vi "Write Data.vi"(7 "Address":u16=65535 format="%.0x", 8 "error in (no error)":errorcluster, 9 "Data":i32[](array[numeric]), 10 "Specified Num in":u8=1, 11 "Port Selection Info":T1={"Port Name"="", "Amplifier Num"=1, "Baud Rate"=38400, "Char Formation"=enum."0"} {"Baud Rate" items=["38400"=38400, "19200"=19200, "9600"=9600, "115200"=0]; "Amplifier Num" max=31}) -> (0 "error out":errorcluster, 2 "Specified Num out":u8=1, 3 "Port Selection Info Out":T1={"Port Name"="", "Amplifier Num"=1, "Baud Rate"=38400, "Char Formation"=enum."0"} {"Baud Rate" items=["38400"=38400, "19200"=19200, "9600"=9600, "115200"=0]; "Amplifier Num" max=31})   [LabVIEW 2014, in "ALPHA5 RS485.lvlib"]
uses:
  ALPHA5 RS485.lvlib
  typedefs/Port Selection Info.ctl
panel:
  # "FC: 10h\nWrite Data of Different Types"
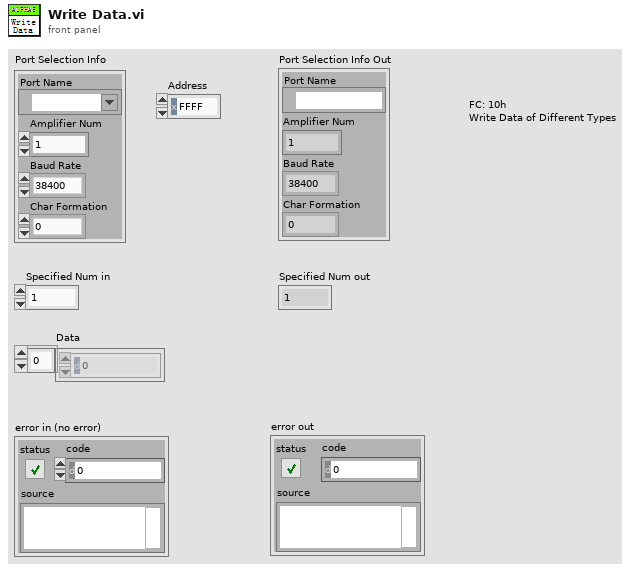
[diagram p1: front panel]
types:
  T1 = typedef "ALPHA5 RS485.lvlib/Port Selection Info.ctl" = cluster{"Port Name":refnum<visa-resource-name>, "Amplifier Num":u8, "Baud Rate":u32, "Char Formation":enum16{"0", "1", "2", "3", "4", "5"}}
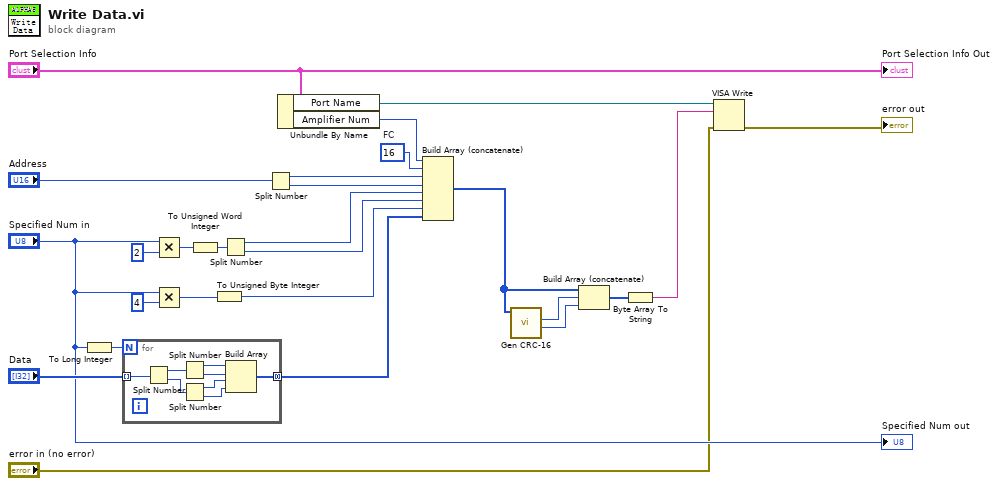
[diagram p0: block diagram]
diagram:
  w17 = u8 16  # FC
  n1 = To Long Integer(number="Specified Num in") -> (32bit integer=w5:i32)
  n2 = for {
    N: w5 -> [_]
    tunnel: "Data" -> [w34] mode=indexing
    tunnel: [w28] -> w4 mode=concatenating
    n3 = Split Number(x=w34) -> (hi(x)=w33:u16, lo(x)=w32:u16)
    n4 = Split Number(x=w33) -> (hi(x)=w31:u8, lo(x)=w30:u8)
    n5 = Split Number(x=w32) -> (hi(x)=w29:u8, lo(x)=w27:u8)
    n6 = Build Array(w31, w30, w29, w27) -> (w28:u8[])
  }
  n7 = Multiply(x="Specified Num in", y=u8 2) -> (x*y=w13:u8)
  n8 = Multiply(x="Specified Num in", y=u8 4) -> (x*y=w8:u8)
  n9 = To Unsigned Word Integer(number=w13) -> (unsigned 16bit integer=w12:u16)
  n10 = To Unsigned Byte Integer(number=w8) -> (unsigned 8bit integer=w7:u8)
  n11 = Split Number(x=w12) -> (hi(x)=w11:u8, lo(x)=w10:u8)
  n12 = Split Number(x="Address") -> (hi(x)=w16:u8, lo(x)=w15:u8)
  n13 = Unbundle By Name("Port Selection Info") -> ("Port Name"=w19:refnum<visa-resource-name>, "Amplifier Num"=w24:u8)
  n14 = Build Array (concatenate)(w24, w17, w16, w15, w11, w10, w7, w4) -> (w20:u8[])
  n15 = call "Gen CRC-16.vi"("Data In"=w20) -> ("CRC-16-H"=w22:u8, "CRC-16-L"=w23:u8)  [unwired: 7 in, 2 out]
  n16 = Build Array (concatenate)(w20, w23, w22) -> (w21:u8[])
  n17 = Byte Array To String(unsigned byte array=w21) -> (string=w18:string)
  n18 = VISA Write(VISA resource name=w19, write buffer=w18, error in (no error)="error in (no error)") -> (error out=→"error out":errorcluster)  [unwired: 2 out]
  "Port Selection Info Out" <- "Port Selection Info"
  "Specified Num out" <- "Specified Num in"
